vi "UDP.Rx.vi"(5 "max size (548)":i32=548, 7 "port":u16=60000, 8 "error in (no error)":errorcluster, 10 "Count Pointer":refnum<class "Pointer.lvclass">, 11 "Stop Pointer":refnum<class "Pointer.lvclass">) -> (0 "error out":errorcluster)   [LabVIEW 2017]
uses:
  <vilib>/NI/Memory Manager/Classes/Pointer/Pointer.lvclass
  <vilib>/NI/Memory Manager/Classes/Pointer/Pointer.lvclass/Pointer.ctl
  <vilib>/NI/Memory Manager/Classes/Pointer/Public/Write/Write (0D I32).vi
  <vilib>/NI/Memory Manager/Classes/Pointer/Public/Read/Read (0D Bool).vi
  <vilib>/NI/Memory Manager/Classes/Pointer/Public/Write/Write (0D Bool).vi
  <vilib>/NI/Memory Manager/Classes/Pointer/Public/Write (No Check)/Write (No Check 0D I32).vi
  <vilib>/NI/Memory Manager/Classes/Pointer/Protected/Parameter Checking/Check Null Pointer.vi
  <vilib>/NI/Memory Manager/Classes/Pointer/Protected/Parameter Checking/Check Subset.vi
  <vilib>/NI/Memory Manager/Classes/Pointer/Public/Read (No Check)/Read (No Check 0D Bool).vi
  <vilib>/NI/Memory Manager/Classes/Pointer/Public/Write (No Check)/Write (No Check 0D Bool).vi
  <vilib>/NI/Memory Manager/Classes/Pointer/API/Accessors/Get Address.vi
  <vilib>/NI/Memory Manager/Classes/Pointer/Protected/Errors.vi
  <vilib>/NI/Memory Manager/Classes/Pointer/Protected/Error VIs/Null Pointer.vi
  <vilib>/NI/Memory Manager/Classes/Pointer/Protected/Error VIs/Out of Bounds.vi
  <vilib>/NI/Memory Manager/Classes/Pointer/API/Accessors/Get Size.vi
  <vilib>/NI/Memory Manager/Classes/Pointer/Protected/Error Building/Create Error.vi
  <vilib>/NI/Memory Manager/VIs/Write String into Source.vi
  <vilib>/NI/Memory Manager/Classes/Pointer/Protected/Error Building/Write Pointer Size.vi
  <vilib>/NI/Memory Manager/VIs/Write Number into Source.vi
  <vilib>/NI/Memory Manager/VIs/VIs for Poly/Write U64 into Source.vi
  <vilib>/NI/Memory Manager/Constants/Constants.vi
  <vilib>/NI/Memory Manager/Constants/Library Name.vi
  <vilib>/NI/Memory Manager/Classes/Pointer/Protected/Error Building/Get Error Info.vi
  <vilib>/NI/Memory Manager/VIs/Create Error Cluster.vi
  <vilib>/NI/Memory Manager/VIs/VIs for Poly/Create Error Cluster (256B).vi
  <vilib>/NI/Memory Manager/VIs/Set Error Status.vi
  <vilib>/NI/Memory Manager/VIs/Set Error Code.vi
  <vilib>/NI/Memory Manager/VIs/Set Error Source.vi
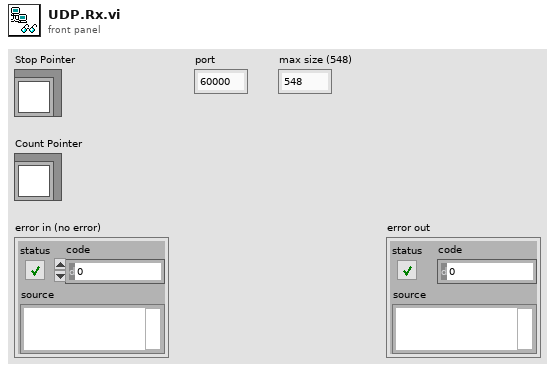
[diagram p1: front panel]
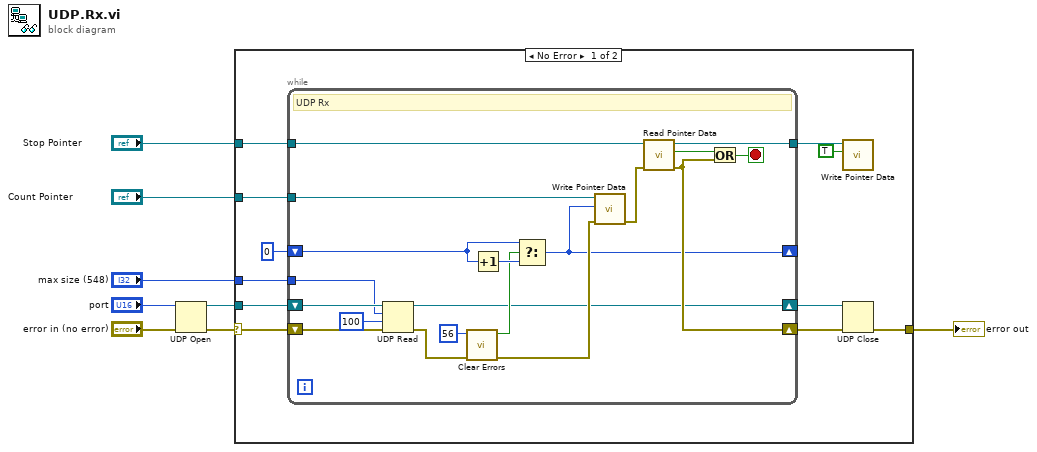
[diagram p0: block diagram]
diagram:
  n1 = UDP Open(8:"error in (no error)", 11:"port") -> (port=w8:refnum<k16>, 0:w2:errorcluster)  [unwired: 3 in, 1 out]
  n2 = case shown="No Error" w2 {
    selector: w2 -> [w12 w39]
    tunnel: w8 -> [w19 _]
    tunnel: "max size (548)" -> [w18 _]
    tunnel: "Stop Pointer" -> [w16 _]
    tunnel: "Count Pointer" -> [w15 _]
    tunnel: [w9 w39] -> w1
    frame No Error {
      n3 = while {
        shift-right: [w23] -> w11
        shift-left: w12 -> [w37]
        shift-right: [w22] -> w10
        shift-left: w19 -> [w38]
        tunnel: w16 -> [w29]
        tunnel: w18 -> [w35]
        shift-right: [w20] -> _
        shift-left: 0 -> [w31]
        tunnel: w15 -> [w27]
        tunnel: [w21] -> w14
        stop <- w36 stop-if-true
        # "UDP Rx"
        n4 = UDP Read(connection ID=w38, max size (548)=w35, timeout ms (25000)=100, 8:w37) -> (error out=w32:errorcluster, 3:w22:refnum<k16>)  [unwired: 3 out]
        n5 = call <vilib>:"Clear Errors.vi"("error in (no error)"=w32, "specific error code to clear (0: all)"=56) -> ("error out"=w25:errorcluster, "specific error cleared?"=w28:bool)  [unwired: 4 in]
        n6 = Increment(x=w31) -> (x+1=w30:i32)
        n7 = Select(t=w31, s=w28, f=w30) -> (s? t:f=w20:i32)
        n8 = call-poly <vilib>:"Write Pointer Data.vi"("error in (no error)"=w25, "value"=w20, "Pointer in"=w27) -> ("error out"=w24:errorcluster)  [unwired: 5 in, 3 out]
        n9 = call-poly <vilib>:"Read Pointer Data.vi"("error in (no error)"=w24, "Pointer in"=w29) -> ("error out"=w23:errorcluster, "value out"=w26:bool, "Pointer out"=w21:refnum<class "Pointer.lvclass">)  [unwired: 6 in, 1 out]
        n10 = Or(x=w26, y=w23) -> (x .or. y?=w36:bool)
      }
      n11 = call-poly <vilib>:"Write Pointer Data.vi"("value"=TRUE, "Pointer in"=w14) -> ()  [unwired: 6 in, 4 out]
      n12 = UDP Close(connection ID=w10, 8:w11) -> (error out=w9:errorcluster)  [unwired: 1 out]
    }
    frame Error {
    }
  }
  "error out" <- w1
